vi "G#Object_IsCallerMethodOfSameClass.vi"(3 "call depth (1)":i32=1, 5 "reference in":refnum<class "G#Object.lvclass">) -> (0 "reference full class name":string, 1 "is caller of G#Object?":bool, 2 "is of same class?":bool)   [LabVIEW 2020, in "G#Object.lvclass"]
doc: "Checks if caller method specified by the call depth is of same class as the run-time input reference."
uses:
  <vilib>/addons/_AddQ/G#Object/G#Object.lvclass
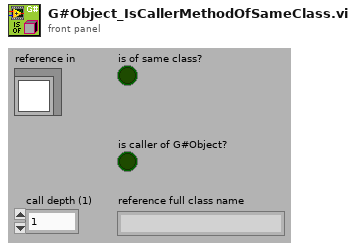
[diagram p1: front panel]
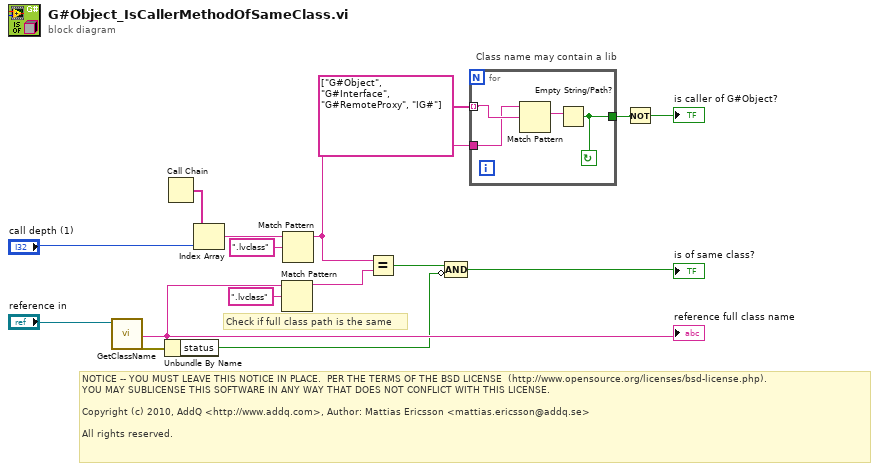
[diagram p0: block diagram]
diagram:
  # "Class name may contain a lib"
  # "NOTICE -- YOU MUST LEAVE THIS NOTICE IN PLACE.  PER THE TERMS OF THE BSD LICENSE  (http://www.opensource.org/licenses/bsd-license.php).\nYOU MAY SUBLICENSE THIS SOFTWARE IN ANY WAY THAT DOES NOT CONFLICT WITH THIS LICENSE.\n\nCopyright (c) 2010, AddQ <http://www.addq.com>, Author: Mattias Ericsson <mattias.ericsson@addq.se>\n\nAll rights reserved."
  # "Check if full class path is the same"
  n1 = call-dynamic "GetClassName.vi"("reference in"="reference in") -> ("full class name"=w13:string, "error out"=w10:errorcluster)  [unwired: 14 in, 3 out]
  "reference full class name" <- w13
  n2 = Unbundle By Name(w10) -> ("status"=w8:bool)
  n3 = Call Chain() -> (call chain=w11:string[])
  n4 = Index Array(array=w11, index="call depth (1)") -> (element=w5:string)
  n5 = Match Pattern(string=w13, regular expression=".lvclass") -> (before substring=w12:string)  [unwired: 1 in, 3 out]
  n6 = Match Pattern(string=w5, regular expression=".lvclass") -> (before substring=w3:string)  [unwired: 1 in, 3 out]
  n7 = Equal?(x=w3, y=w12) -> (x = y?=w9:bool)
  n8 = Compound Arithmetic op=AND(w9, invert w8) -> (→"is of same class?":bool)
  n9 = for {
    tunnel: string[] ["G#Object", "G#Interface", "G#RemoteProxy", "IG#"] -> [w18] mode=indexing
    tunnel: w3 -> [w17]
    tunnel: [w19] -> w2
    stop <- w19 continue-if-true
    n10 = Match Pattern(string=w17, regular expression=w18) -> (match substring=w20:string)  [unwired: 1 in, 3 out]
    n11 = Empty String/Path?(string/path=w20) -> (empty?=w19:bool)
  }
  n12 = Not(x=w2) -> (.not. x?=→"is caller of G#Object?":bool)
